vi "Check Loop Error.vi"(9 "忽略错误":i32[](array[numeric]), 10 "待处理的错误":cluster{"状态":bool, "代码":i32, "源":string}, 11 "消息队列":refnum<queue>) -> (2 "错误入队列？":bool, 3 "消息队列副本":refnum<queue>)   [LabVIEW 2018]
doc: "检查“待处理消息”的代码是否与“忽略错误”数组中的任意一项匹配。如存在匹配，则不做处理。如不存在匹配，则向“消息处理循环”发送包含错误数据的Error消息，以便对错误进一步处理。"
uses:
  Message Queue/Message Cluster.ctl
  Message Queue/Enqueue Message (Single).vi
  Message Queue/Message Queue.lvlib
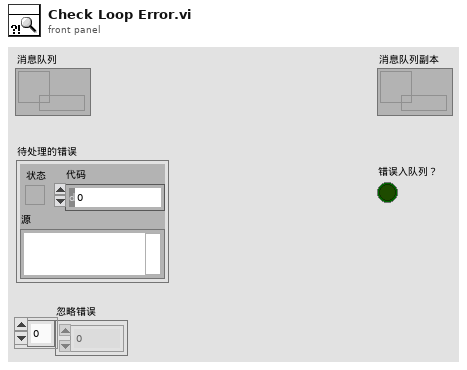
[diagram p1: front panel]
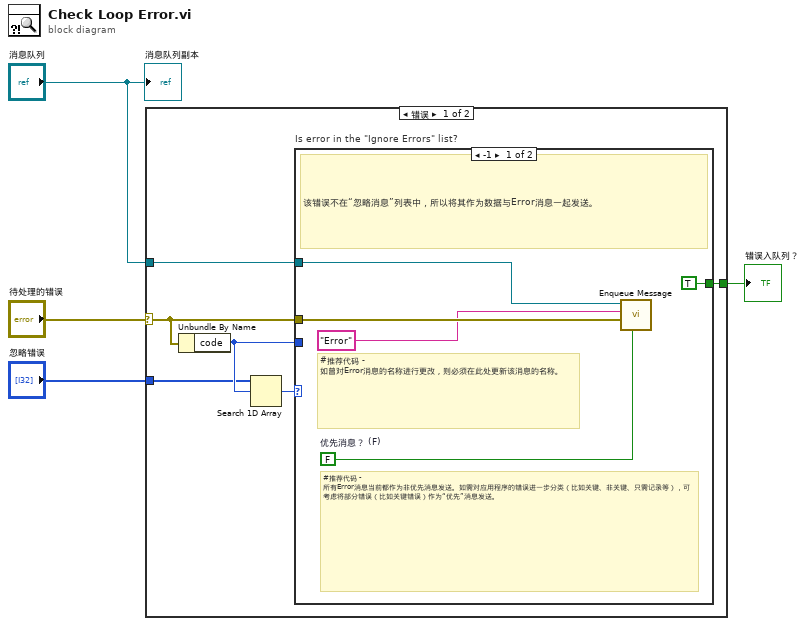
[diagram p0: block diagram]
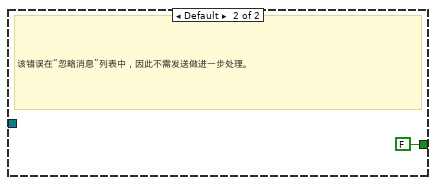
[diagram p2: hidden frame]
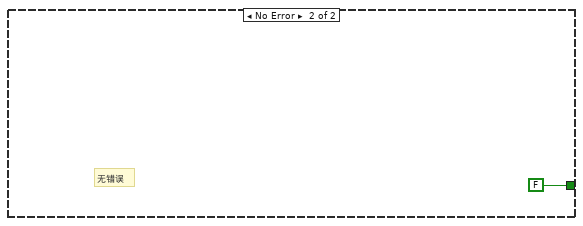
[diagram p3: hidden frame]
diagram:
  n1 = case shown="错误" "待处理的错误" {
    selector: "待处理的错误" -> [w7 _]
    tunnel: "消息队列" -> [w10 _]
    tunnel: "忽略错误" -> [w6 _]
    tunnel: [w5 FALSE] -> w1
    frame Error {
      n2 = Unbundle By Name(w7) -> ("code"=w8:i32)
      n3 = Search 1D Array(1D array=w6, element=w8) -> (index of element=w9:i32)  [unwired: 1 in]
      n4 = case "Is error in the \"Ignore Errors\" list?" shown="-1" w9 {
        tunnel: w7 -> [w13 _]
        tunnel: w10 -> [w15 _]
        tunnel: w8 -> [_ _]
        tunnel: [TRUE FALSE] -> w5
        frame -1 {
          w11 = FALSE  # 优先消息？ (F)
          # "#推荐代码 - 所有Error消息当前都作为非优先消息发送。如需对应用程序的错误进一步分类（比如关键、非关键、只需记录等），可考虑将部分错误（比如关键错误）作为“优先”消息发送。"
          # "#推荐代码 - 如曾对Error消息的名称进行更改，则必须在此处更新该消息的名称。"
          # "该错误不在“忽略消息”列表中，所以将其作为数据与Error消息一起发送。"
          n5 = call-poly "Enqueue Message.vi"("优先消息？ (F)"=w11, "消息数据"=w13, "消息"="Error" ("Message"), "消息队列"=w15) -> ()  [unwired: 6 in, 2 out]
        }
        frame Default {
          # "该错误在“忽略消息”列表中，因此不需发送做进一步处理。"
        }
      }
    }
    frame No Error {
      # "无错误"
    }
  }
  "错误入队列？" <- w1
  "消息队列副本" <- "消息队列"
